vi "Open Form.vi"(8 "error in (no error)":errorcluster, 10 "Panel Form Controller":refnum<class "Panel Form Controller.lvclass">, 11 "Form Model in":refnum<class "Form Model.lvclass">) -> (0 "error out":errorcluster, 3 "Form Model out":refnum<class "Form Model.lvclass">)   [LabVIEW 2020, in "Form Model.lvlib" / "Form Model.lvclass"]
uses:
  Form Model.lvclass
  C:/Program Files (x86)/National Instruments/LabVIEW 2020/vi.lib/ActorFramework/Actor/Actor.lvclass
  Form Controller/Panel Form Controller.lvclass
  <vilib>/ActorFramework/Actor/Actor.lvclass/Actor.ctl
  Form Model.lvclass/Form Model.ctl
  Form Server Messages Messages/Open Form Msg/Open Form Msg.lvclass/Open Form Msg.ctl
  <vilib>/ActorFramework/Message Enqueuer/Message Enqueuer.lvclass/Message Enqueuer.ctl
  <vilib>/ActorFramework/Message Enqueuer/Enqueue.vi
  Form Server Messages Messages/Open Form Msg/Open Form Msg.lvclass
  C:/Program Files (x86)/National Instruments/LabVIEW 2020/vi.lib/ActorFramework/Message/Message.lvclass
  <vilib>/ActorFramework/Message Priority Queue/Priority Enqueue.vi
  Form Configuration/Form Model Configuration.lvclass
  <vilib>/ActorFramework/Actor/Actor.lvclass
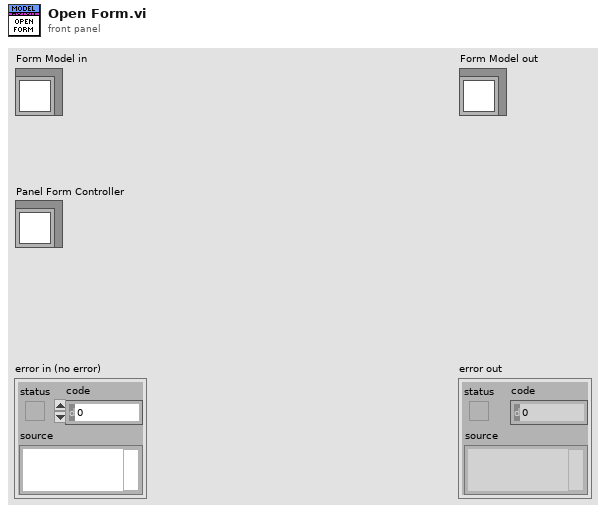
[diagram p1: front panel]
types:
  T1 = typedef "Form Server Interfaces.lvlib/Form ID.ctl" = cluster{"Name":string, "Panel type":string}
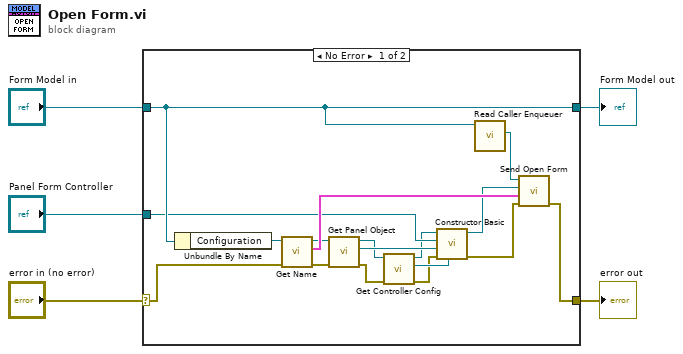
[diagram p0: block diagram]
diagram:
  n1 = case shown="No Error" "error in (no error)" {
    selector: "error in (no error)" -> [w7 w24]
    tunnel: "Form Model in" -> [w22 w23]
    tunnel: [w6 w24] -> w3
    tunnel: [w22 w23] -> w2
    tunnel: "Panel Form Controller" -> [w15 _]
    frame No Error {
      n2 = Unbundle By Name(w22) -> ("Configuration"=w20:refnum<class "Form Model Configuration.lvclass">)
      n3 = call-dynamic "Get Name.vi"("error in (no error)"=w7, "Form Configuration in"=w20) -> ("error out"=w9:errorcluster, "Form ID"=w19:T1, "Form Configuration out"=w14:refnum<class "Form Model Configuration.lvclass">)  [unwired: 7 in]
      n4 = call-dynamic "Get Panel Object.vi"("error in (no error)"=w9, "Form Model Configuration in"=w14) -> ("error out"=w10:errorcluster, "Panel"=w16:refnum<class "Panel.lvclass">, "Form Model Configuration out"=w13:refnum<class "Form Model Configuration.lvclass">)  [unwired: 7 in]
      n5 = call-dynamic "Get Controller Config.vi"("error in (no error)"=w10, "Form Model Configuration in"=w13) -> ("error out"=w11:errorcluster, "Controller config"=w17:refnum<class "Panel Form Controller Configuration.lvclass">, "Form Model Configuration out"=w12:refnum<class "Form Model Configuration.lvclass">)  [unwired: 7 in]
      n6 = call "Constructor Basic.vi"("Controller Config"=w17, "error in (no error)"=w11, "Panel"=w16, "Panel Form Controller"=w15, "Form Model Configuration in"=w12) -> ("error out"=w8:errorcluster, "Form Model Configuration out"=w18:refnum<class "Form Model Configuration.lvclass">)  [unwired: 5 in]
      n7 = call <vilib>:"Read Caller Enqueuer.vi"("Actor"=w22) -> ("Caller Enqueuer"=w21:refnum<class "Message Enqueuer.lvclass">)  [unwired: 10 in]
      n8 = call "Send Open Form.vi"("error in (no error)"=w8, "Caller Name"=w19, "Form Config"=w18, "Message Enqueuer"=w21) -> ("error out"=w6:errorcluster)  [unwired: 6 in, 1 out]
    }
    frame Error {
    }
  }
  "error out" <- w3
  "Form Model out" <- w2
